vi "Get Answers Data.vi"(8 "error in (no error)":errorcluster, 10 "data":u32, 11 "length":u32) -> (0 "error out":errorcluster, 2 "data out":u32, 3 "function return":bool)   [LabVIEW 2015, in "XGL_DPP.lvlib"]
doc: "EXTERN DECLSPEC bool CALL_CONV GetAnswersData(uint32_t length, uint32_t * data);"
uses:
  XGL_DPP.lvlib
  XGL_DPP.dll
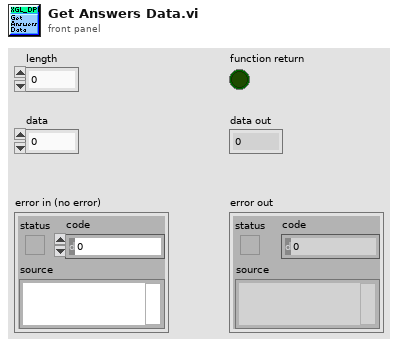
[diagram p1: front panel]
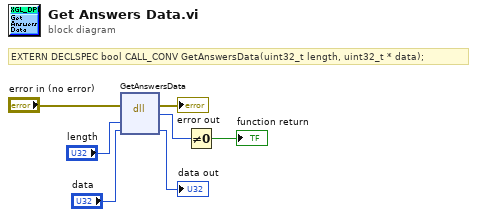
[diagram p0: block diagram]
diagram:
  # "EXTERN DECLSPEC bool CALL_CONV GetAnswersData(uint32_t length, uint32_t * data);"
  n1 = dll-call lib="D:/Users/XRF/Desktop/Scanning Software_Demokritos_2015_v7/libs/Vis_2/XGL_DPP.*" fn="GetAnswersData"(error in="error in (no error)", "length"="length", "data"="data") -> (error out=→"error out":errorcluster, w6:u8, "data"=→"data out":u32)  [unwired: 3 in, 1 out]
  n2 = Not Equal To 0?(x=w6) -> (x != 0?=→"function return":bool)
